vi "Subscribe.vi"(8 "error in (no error)":errorcluster, 10 "Topic":string, 11 "MQTT1 in":refnum<class "MQTT1.lvclass">) -> (0 "error out":errorcluster, 3 "MQTT1 out":refnum<class "MQTT1.lvclass">)   [LabVIEW 2017, in "MQTT1.lvclass"]
uses:
  MQTT1.lvclass
  Libraries/mqtt Folder/src/class/mqtt/mqttTypedef/mqttSubscribeCluster.ctl
  Libraries/mqtt Folder/src/class/mqtt/mqttTypedef/mqttQOSlevel.ctl
  Libraries/mqtt Folder/src/class/mqtt/mqtt.lvclass
panel:
  out "success":bool
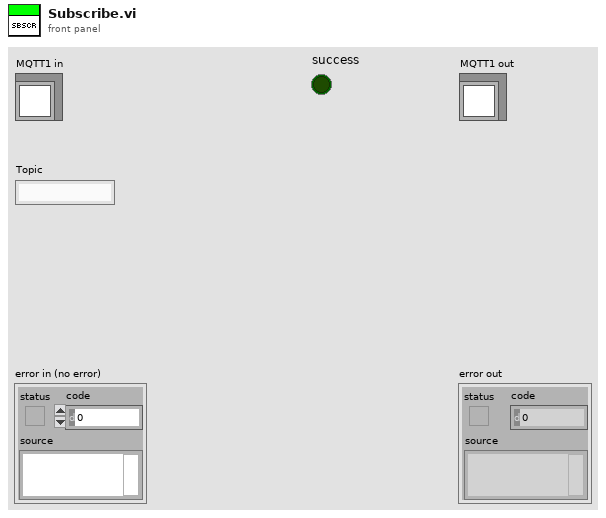
[diagram p1: front panel]
types:
  T1 = typedef "mqttSubscribeCluster.ctl" = cluster{"Topic":string, "QoS":T2}
  T2 = typedef "mqttQOSlevel.ctl" = enum8{"At most once", "At least once", "Exactly once", "Reserved"}
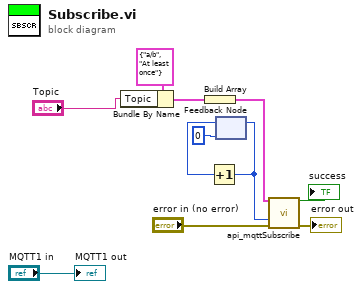
[diagram p0: block diagram]
diagram:
  n1 = Bundle By Name(cluster=T1 {"Topic"="a/b", "QoS"=enum."At least once"} ("Subscription Info"), "Topic"="Topic") -> (w7:T1)
  n2 = Build Array(w7) -> (w6:T1[])
  n3 = feedback #1(u16 0) -> (w3:u16)
  n4 = Increment(x=w3) -> (x+1=w2:u16)
  n5 = feedback-in #1(w2) -> ()
  n6 = call "api_mqttSubscribe.vi"("subscriptionInfo"=w6, "messageID"=w2, "error in (no error)"="error in (no error)") -> ("success"=→"success":bool, "error out"=→"error out":errorcluster)  [unwired: 11 in]
  "MQTT1 out" <- "MQTT1 in"
